vi "Acquire voltage waveform.vi"(0 "Connection ID":refnum<k5>, 5 "channel index":i8, 9 "method":T1={"sampling interval"=0.1, "samples to average"=1, "data interval"=0.0, "stream data"=FALSE, "file path"=refnum, "command"={"command"=enum."Idle", "start time (ms)"=0, "Channel Indices"=[], "Scans per Sample"=1}} {"command"."Scans per Sample" min=1; "data interval" format="%.2f"; "samples to average" min=1 step=1; "sampling interval" format="%.2f"}, 11 "data points to acquire":u32=1000 min=1) -> (4 "Connection ID out":refnum<k5>, 6 "channel data array":sgl[](array[numeric]) format="%.5f", 8 "mean":dbl format="%.2f", 10 "cv":dbl format="%.2f", 14 "canceled":bool, 15 "all data":sgl[][](array[numeric]) format="%.5f")   [LabVIEW 2012]
uses:
  DAC apps/support/method.ctl
  DataServer/command cluster.ctl
  DataServer/command.ctl
  <vilib>/Analysis/NI_AALBase.lvlib
panel:
  out "Array display to eliminate reshape bug":sgl[](array[numeric]) format="%.2f"
  in  "Monitoring sample":bool
  out "chart":sgl[](graph)
  # "s"
  # "s"
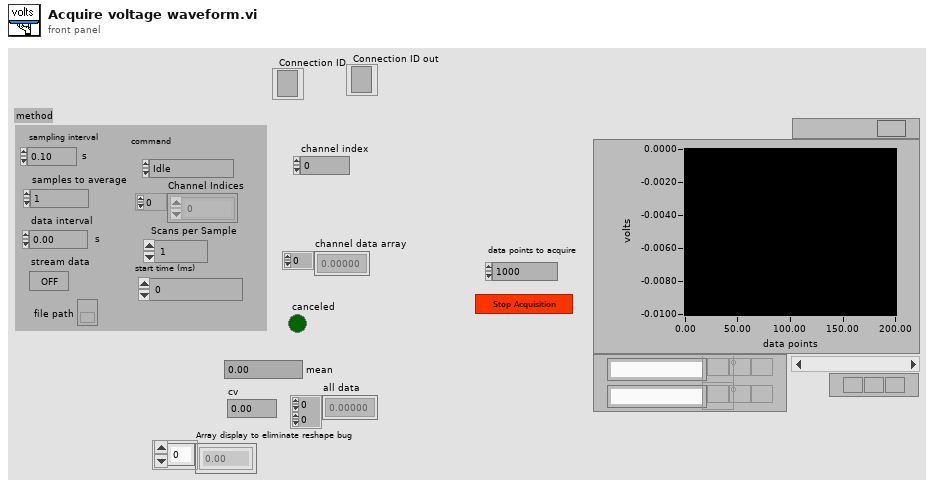
[diagram p1: front panel]
types:
  T1 = typedef "method.ctl" = cluster{"sampling interval":sgl, "samples to average":u32, "data interval":sgl, "stream data":bool, "file path":refnum<file>, "command":T2}
  T2 = typedef "command cluster.ctl" = cluster{"command":T3, "start time (ms)":u32, "Channel Indices":i32[], "Scans per Sample":i32}
  T3 = typedef "command.ctl" = enum16{"Idle", "Send Data", "Send 1 Scan", "Logoff"}
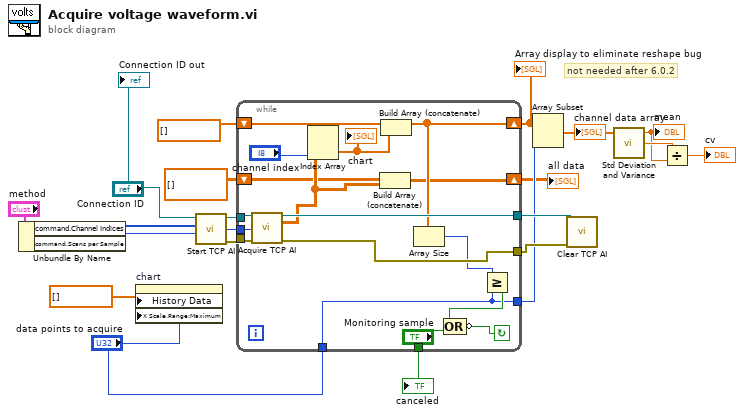
[diagram p0: block diagram]
diagram:
  # "not needed after 6.0.2"
  n1 = Unbundle By Name("method") -> ("command.Channel Indices"=w6:i32[], "command.Scans per Sample"=w5:i32)
  n2 = property on="chart" class="WFChart (strict)"("History Data"=sgl[] [], "X Scale.Range:Maximum"="data points to acquire") -> ()  [unwired: 2 in, 2 out]
  n3 = call "Start TCP AI.vi"("Scans per Sample"=w5, "channel indices"=w6, "Connection ID in"="Connection ID") -> ("error out"=w20:errorcluster, "channels"=w19:i32, "Connection ID out"=w18:refnum<k5>)  [unwired: 6 in]
  n4 = while {
    shift-left: sgl[][] [] -> [w23]
    shift-right: [w22] -> w2
    tunnel: "data points to acquire" -> [w27]
    tunnel: [w27] -> w4
    tunnel: ["Monitoring sample"] -> w12
    tunnel: [w30] -> w16
    tunnel: w19 -> [w31]
    shift-left: sgl[] [] -> [w35]
    shift-right: [w28] -> w10
    tunnel: w18 -> [w34]
    tunnel: [w32] -> w17
    tunnel: w20 -> [w33]
    stop <- w38 continue-if-true
    n5 = call "Acquire TCP AI.vi"("connection ID"=w34, "channels"=w31, "error in"=w33) -> ("connection ID out"=w30:refnum<k5>, "voltage data"=w24:sgl[][], "error out"=w32:errorcluster)  [unwired: 8 in, 2 out]
    n6 = Index Array(array=w24, index (col)="channel index") -> (element=w25:sgl[])  [unwired: 1 in]
    "chart" <- w25
    n7 = Build Array (concatenate)(w23, w24) -> (w22:sgl[][])
    n8 = Build Array (concatenate)(w35, w25) -> (w28:sgl[])
    n9 = Array Size(array=w28) -> (size(s)=w29:i32)
    n10 = Greater Or Equal?(x=w29, y=w27) -> (x >= y?=w36:bool)
    n11 = Compound Arithmetic op=OR(w36, "Monitoring sample") -> (invert w38:bool)
  }
  "canceled" <- w12
  "all data" <- w2
  "Array display to eliminate reshape bug" <- w10
  n12 = Array Subset(array=w10, length=w4) -> (w11:sgl[])  [unwired: 1 in]
  "channel data array" <- w11
  n13 = call "Clear TCP AI.vi"("error in (no error)"=w17, "Connection ID in"=w16) -> ()  [unwired: 8 in, 2 out]
  n14 = call <vilib>:"Std Deviation and Variance.vi"("X"=w11) -> ("mean"=w14:dbl, "standard deviation"=w15:dbl)  [unwired: 1 in, 1 out]
  "mean" <- w14
  n15 = Divide(x=w15, y=w14) -> (x/y=→"cv":dbl)
  "Connection ID out" <- "Connection ID"
